vi "Enable Wash Steps.vi"(8 "error in (no error)":errorcluster, 10 "Disabled":T1(ring), 11 "Sim Entry Console Actor in":refnum<class "Sim Entry Console Actor.lvclass">) -> (0 "error out":errorcluster, 3 "Sim Entry Console Actor out":refnum<class "Sim Entry Console Actor.lvclass">)   [LabVIEW 2019, in "Sim Entry Console Actor.lvlib" / "Sim Entry Console Actor.lvclass"]
uses:
  Sim Entry Console Actor.lvclass
  Sim Entry Console Actor.lvclass/Sim Entry Console Actor.ctl
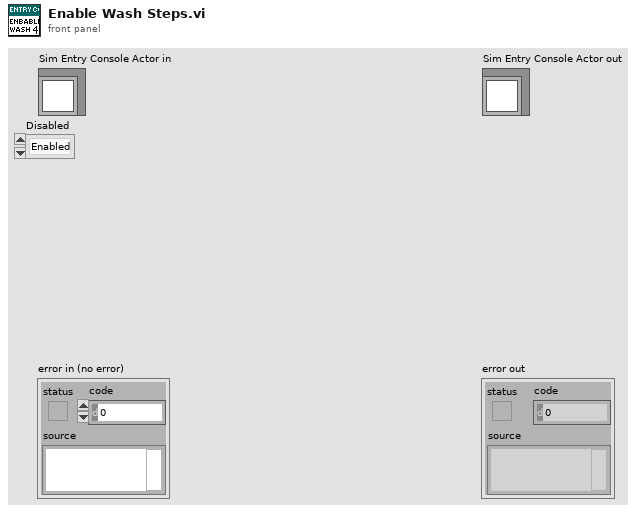
[diagram p1: front panel]
types:
  T1 = enum8{"Enabled", "Disabled", "Disabled and Grayed Out"}
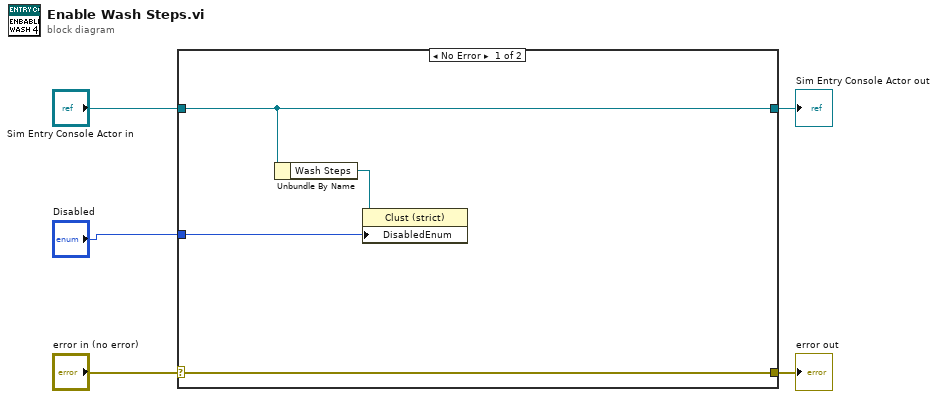
[diagram p0: block diagram]
diagram:
  n1 = case shown="No Error" "error in (no error)" {
    selector: "error in (no error)" -> [w9 w11]
    tunnel: [w9 w11] -> w4
    tunnel: [w8 w10] -> w2
    tunnel: "Sim Entry Console Actor in" -> [w8 w10]
    tunnel: "Disabled" -> [w6 _]
    frame No Error {
      n2 = Unbundle By Name(w8) -> ("Wash Steps"=w7:refnum<vi>)
      n3 = property class="Clust (strict)"(reference=w7, "DisabledEnum"=w6) -> ()  [unwired: 1 in, 2 out]
    }
    frame Error {
    }
  }
  "error out" <- w4
  "Sim Entry Console Actor out" <- w2
